vi "QueryServer_Event_Add.vi"(7 "server id":i32, 8 "error in (no error)":errorcluster, 9 "status":i32, 10 "eventdata":string, 11 "gRPCid":T2) -> (0 "error out":errorcluster, 3 "gRPCid out":T2)   [LabVIEW 2019]
uses:
  QueryServer_gRPCid.ctl
  QueryServer_Event.ctl
  Debug/labview_query_server.dll
panel:
  in  "ServerEvent":T1
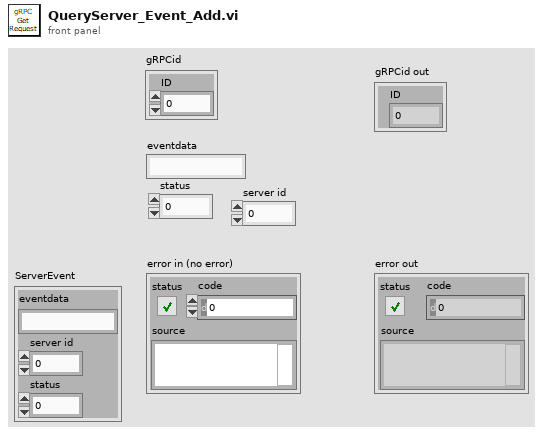
[diagram p1: front panel]
types:
  T1 = typedef "QueryServer_Event.ctl" = cluster{"eventdata":string, "server id":i32, "status":i32}
  T2 = typedef "QueryServer_gRPCid.ctl" = cluster{"ID":u64}
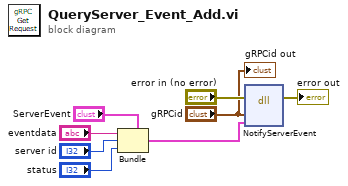
[diagram p0: block diagram]
diagram:
  n1 = Bundle(cluster="ServerEvent", "eventdata"="eventdata", "server id"="server id", "status"="status") -> (w4:T1)
  n2 = dll-call lib="C:/dev/labview-grpc-query-server/Debug/labview_query_server.dll" fn="NotifyServerEvent"(error in="error in (no error)", "id"="gRPCid", "data"=w4) -> (error out=→"error out":errorcluster)  [unwired: 5 in, 1 out]
  "gRPCid out" <- "gRPCid"
